vi "color_pattern_recog_server.vi"() -> ()   [LabVIEW 2014]
uses:
  <vilib>/vision/Image Controls.llb/IMAQ Image.ctl
  <vilib>/vision/NI_Vision_Development_Module.lvlib
  <vilib>/vision/driver/NI_Vision_Acquisition_Software.lvlib
panel:
  out "Number of Matches":i32
  in  "Tab Control":enum32{"Page 1", "Page 2"}(tab)
  out "bytes written":i32
  out "remote address":string
  in  "Port":u16=81 min=1025 step=1
  out "remote port":u16
  in  "Stop":bool
  out "Template":T1(plugin-control)
  in  "Image source":bool
  in  "Controls":enum32{"Page 1", "Page 2"}(tab)
  in  "Template wait":u32=1000
  in  "match wait":u32=10
  in  "Nb of Matches":i32=4
  in  "Match Mode 2":u32(ring) items=["Shift Invariant", "Rotation Invariant"]
  in  "Match Feature Mode":u32(ring) items=["Color and Shape", "Color", "Shape"]
  in  "Color Score Weight":sgl=500.0 min=0 max=1000 format="%.2f"
  in  "Minimum Contrast 2":i32=10
  in  "Color Sensitivity":u32(ring)=2 items=["Low Sensitivity", "Medium Sensitivity", "High Sensitivity"]
  in  "Search Strategy":u32(ring) items=["Conservative", "Balance", "Aggressive", "Very Aggressive"]
  in  "Minimum Score 2":sgl=700.0
  in  "Subpixel Accuracy 2":bool
  in  "File Path":path=path "C:/Users/TMRS/Desktop/image procsseing labview/Pattern matching/FuseBox/fuse01-01.jpg"
  in  "Mode select (template/match)":bool=TRUE
  in  "Template path":path=path "C:/Users/TMRS/Desktop/image procsseing labview/Pattern matching/FuseBox/fuse01-00.jpg"
  out "error":errorcluster
  out "image":T1(plugin-control)
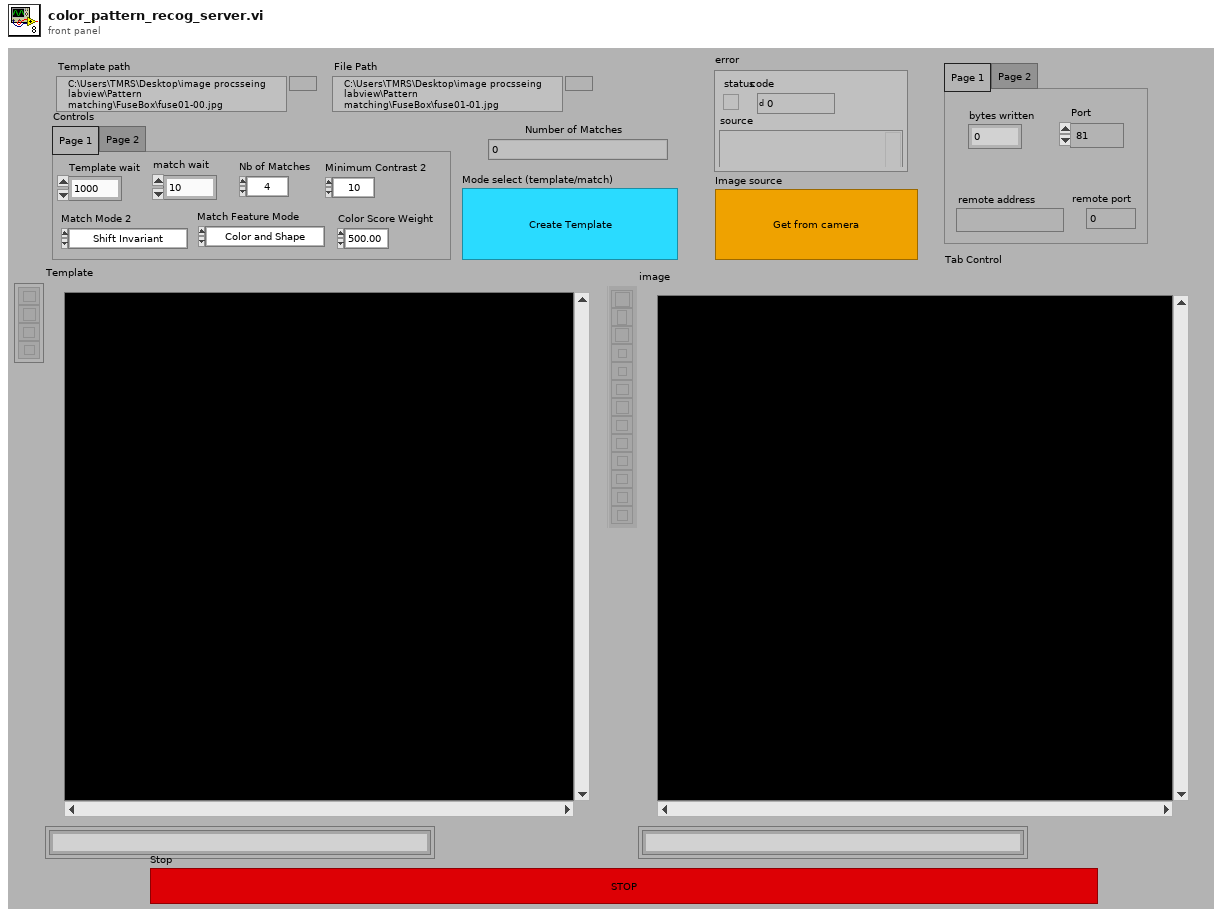
[diagram p1: front panel]
types:
  T1 = typedef "IMAQ Image.ctl" = refnum<image>
  T2 = cluster{"Position":cluster{"x":sgl, "y":sgl}, "Angle":sgl, "Scale":sgl, "Score":sgl, "Bounding Box":cluster{"x":sgl, "y":sgl}[]}[]
  T3 = cluster{"Global Rectangle":i32[], "Contours":cluster{"Contour Type":u32, "ROI Type":u32, "Points":i32[]}[]}
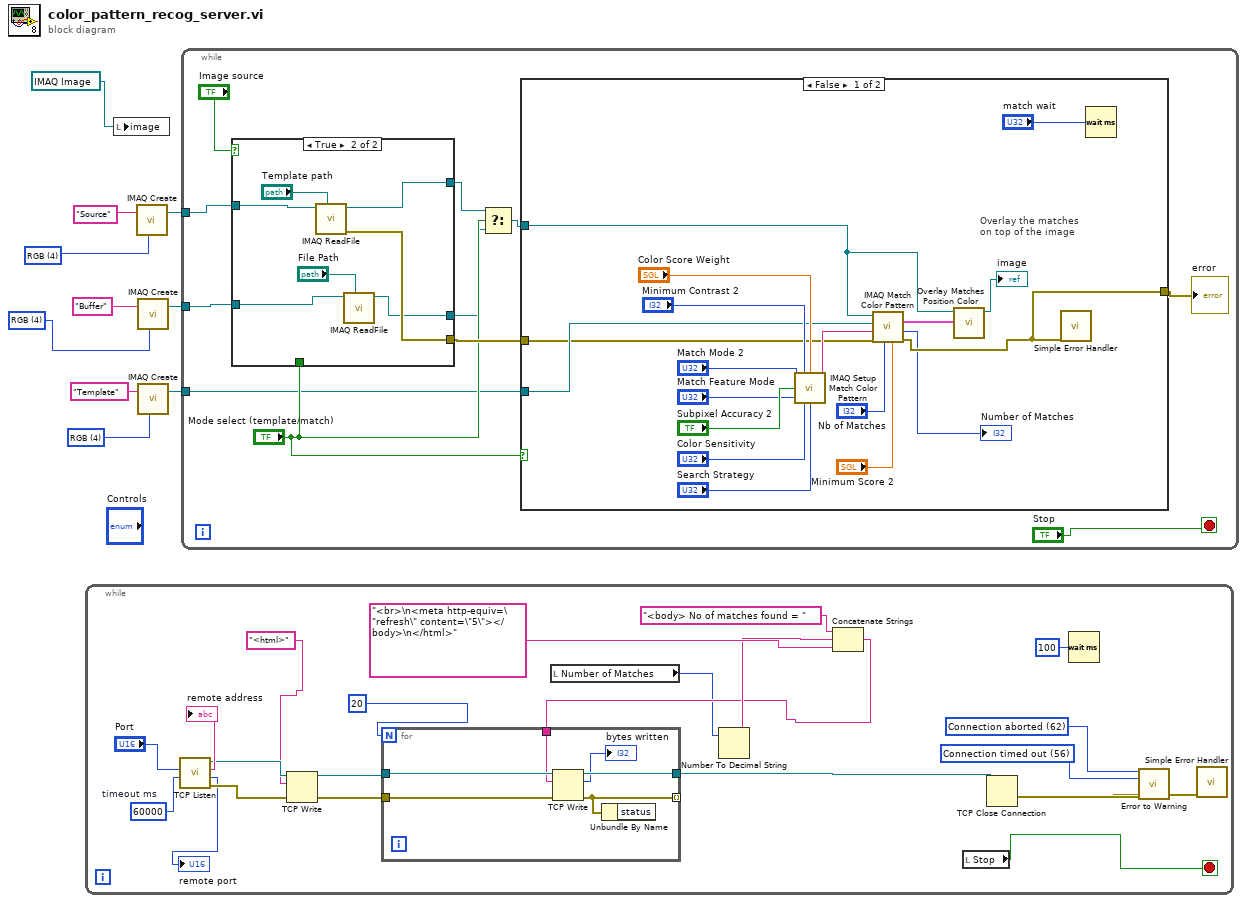
[diagram p0: block diagram]
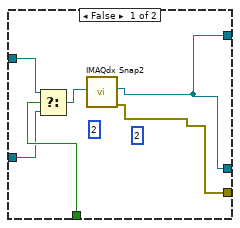
[diagram p2: hidden frame]
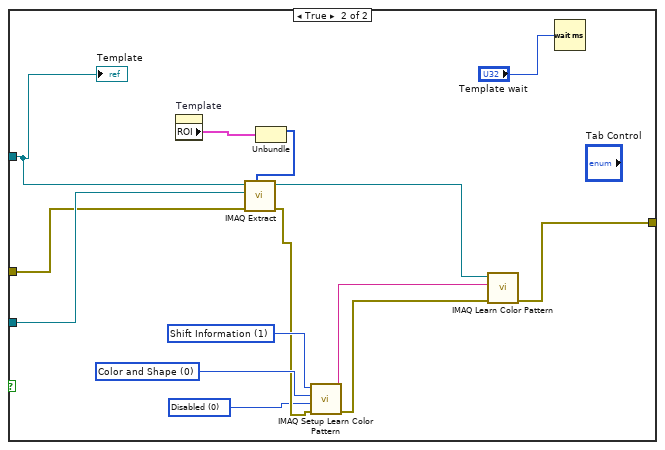
[diagram p3: hidden frame]
diagram:
  w1 = u32 4 items=["8 bits", "16 bits", "Float", "Complex", "RGB", "HSL"] ("Image Type")
  w2 = u32 4 items=["8 bits", "16 bits", "Float", "Complex", "RGB", "HSL"] ("Image Type")
  w3 = u32 4 items=["8 bits", "16 bits", "Float", "Complex", "RGB", "HSL"] ("Image Type")
  n1 = while {
    stop <- w11 stop-if-true
    w26 = 60000  # timeout ms
    w27 = 56 items=["No Error", "Argument Error", "Memory Full", "Out of Zone", "End of File", "File Already Open", "Generic File IO Error", "File Not Found", "File Permission Error", "Disk Full", "Duplicate Path", "Too Many Files Open", "Not Enabled", "Resource File Not Found", "Cannot Add Resource", "Resource Not Found", "Image Not Found", "Image Memory Error", "Pen Does Not Exist", "Config Bad Type", "Config Token Not Found", "Config Parse Error", "Config Memory Error", "Bad External Code Format", "Bad External Code Offset", "External Code Not Present", "Null Window", "Destroy Window Mixup", "Null Menu", "Print Aborted", "Bad Print Record", "Print Driver Error", "Windows Error During Print", "Memory Error During Print", "Print Dialog Error", "Generic Print Error", "Invalid Device Refnum", "Device Not Found", "Device Parameter Error", "Device Unit Error", "Can't Open Device", "Device Call Aborted", "Generic Error", "Cancelled By User", "Object ID Too Low", "Object ID Too High", "Object Not In Heap", "Unknown Heap", "Bad DefProc ID", "DefProc Not In Table", "Message Out Of Range", "Null Method", "Unknown Message", "Manager Call Not Supported", "Bad address", "Connection In progress", "Connection timed out", "Connection is already in progress", "Network attribute not supported", "Network error", "Address in use", "System out of memory", "Connection aborted", "Connection refused", "Connection is not connected", "Connection is already connected", "Connection closed", "Initialize error (interapplication manager)", "Bad occurrence", "Wait on unbound occurrence handler", "Occurrence queue overflow", "Bad path", "Semaphore not signaled", "Unrecognized type (interapplication manager)"] ("2nd Error to Convert")
    w28 = 62 items=["No Error", "Argument Error", "Memory Full", "Out of Zone", "End of File", "File Already Open", "Generic File IO Error", "File Not Found", "File Permission Error", "Disk Full", "Duplicate Path", "Too Many Files Open", "Not Enabled", "Resource File Not Found", "Cannot Add Resource", "Resource Not Found", "Image Not Found", "Image Memory Error", "Pen Does Not Exist", "Config Bad Type", "Config Token Not Found", "Config Parse Error", "Config Memory Error", "Bad External Code Format", "Bad External Code Offset", "External Code Not Present", "Null Window", "Destroy Window Mixup", "Null Menu", "Print Aborted", "Bad Print Record", "Print Driver Error", "Windows Error During Print", "Memory Error During Print", "Print Dialog Error", "Generic Print Error", "Invalid Device Refnum", "Device Not Found", "Device Parameter Error", "Device Unit Error", "Can't Open Device", "Device Call Aborted", "Generic Error", "Cancelled By User", "Object ID Too Low", "Object ID Too High", "Object Not In Heap", "Unknown Heap", "Bad DefProc ID", "DefProc Not In Table", "Message Out Of Range", "Null Method", "Unknown Message", "Manager Call Not Supported", "Bad address", "Connection In progress", "Connection timed out", "Connection is already in progress", "Network attribute not supported", "Network error", "Address in use", "System out of memory", "Connection aborted", "Connection refused", "Connection is not connected", "Connection is already connected", "Connection closed", "Initialize error (interapplication manager)", "Bad occurrence", "Wait on unbound occurrence handler", "Occurrence queue overflow", "Bad path", "Semaphore not signaled", "Unrecognized type (interapplication manager)"] ("1st Error to Convert")
    n2 = call <vilib>:"TCP Listen.vi"("timeout ms (wait forever: -1)"=w26, "port"="Port") -> ("error out"=w25:errorcluster, "remote port"=→"remote port":u16, "remote address"=→"remote address":string, "connection ID"=w20:refnum<k5>)  [unwired: 2 in, 4 out]
    n3 = TCP Write(connection ID=w20, data in="<html>") -> (connection ID out=w21:refnum<k5>)  [unwired: 1 in, 3 out]
    n4 = local read "Number of Matches"() -> (w12:i32)
    n5 = Number To Decimal String(number=w12) -> (decimal integer string=w16:string)  [unwired: 1 out]
    n6 = Concatenate Strings("<body> No of matches found = " ("data in"), w16, "<br>\n<meta http-equiv=\"refresh\" content=\"5\"></body>\n</html>" ("data in")) -> (w15:string)
    n7 = for {
      N: 20 -> [_]
      tunnel: [w37] -> _ mode=indexing
      tunnel: w21 -> [w36]
      tunnel: w25 -> [w35]
      tunnel: [w34] -> w13
      tunnel: w15 -> [w32]
      n8 = TCP Write(connection ID=w36, data in=w32, error in (no error)=w35) -> (connection ID out=w34:refnum<k5>, bytes written=→"bytes written":i32, error out=w37:errorcluster)  [unwired: 1 out]
      n9 = Unbundle By Name(w37) -> ()  [unwired: 1 out]
    }
    n10 = local read "Stop"() -> (w11:bool)
    n11 = TCP Close Connection(connection ID=w13) -> (error out=w30:errorcluster)  [unwired: 1 in, 2 out]
    n12 = Wait (ms)(milliseconds to wait=u32 100) -> ()  [unwired: 1 out]
    n13 = call <vilib>:"Error to Warning.vi"("1st Error to Convert"=w28, "2nd Error to Convert"=w27, "error in"=w30) -> ("warning out"=w29:errorcluster)  [unwired: 3 in, 9 out]
    n14 = call <vilib>:"Simple Error Handler.vi"("error in (no error)"=w29) -> ()  [unwired: 1 in, 8 out]
  }
  n15 = local write "image"(T1 refnum ("Image")) -> ()
  n16 = call "IMAQ Create"("Image Name"="Source", "Image Type"=w2) -> ("New Image"=w8:T1)  [unwired: 2 in, 2 out]
  n17 = call "IMAQ Create"("Image Name"="Buffer" ("Image 3"), "Image Type"=w1) -> ("New Image"=w7:T1)  [unwired: 2 in, 2 out]
  n18 = call "IMAQ Create"("Image Name"="Template", "Image Type"=w3) -> ("New Image"=w9:T1)  [unwired: 2 in, 2 out]
  n19 = while {
    tunnel: w9 -> [w41]
    tunnel: w8 -> [w47]
    tunnel: w7 -> [w45]
    stop <- "Stop" stop-if-true
    n20 = case shown="True" "Image source" {
      tunnel: w47 -> [w52 w61]
      tunnel: [w49 w60] -> w39
      tunnel: [w50 w59] -> w46
      tunnel: w45 -> [w53 w56]
      tunnel: [w49 w55] -> w40
      tunnel: "Mode select (template/match)" -> [w54 _]
      frame False {
        (unwired) 2 ("Step x")
        (unwired) 2 ("Step y")
        n21 = Select(t=w52, s=w54, f=w53) -> (s? t:f=w51:T1)
        n22 = call <vilib>:"IMAQdx Snap2.vi"("Image In"=w51) -> ("error out"=w50:errorcluster, "Image Out"=w49:T1)  [unwired: 8 in, 1 out]
      }
      frame True {
        n23 = call "IMAQ ReadFile"("File Path"="Template path", "Image"=w61) -> ("error out"=w59:errorcluster, "Image Out"=w60:T1)  [unwired: 3 in, 5 out]
        n24 = call "IMAQ ReadFile"("File Path"="File Path", "Image"=w56) -> ("Image Out"=w55:T1)  [unwired: 3 in, 6 out]
      }
    }
    n25 = Select(t=w39, s="Mode select (template/match)", f=w40) -> (s? t:f=w42:T1)
    n26 = case shown="False" "Mode select (template/match)" {
      tunnel: w41 -> [w67 w93]
      tunnel: w46 -> [w62 w91]
      tunnel: [w64 w84] -> w48
      tunnel: w42 -> [w66 w80]
      frame False {
        # "Overlay the matches on top of the image"
        n27 = call "IMAQ Setup Match Color Pattern"("Match Mode"="Match Mode 2", "Minimum Contrast"="Minimum Contrast 2", "Color Score Weight"="Color Score Weight", "Match Feature Mode"="Match Feature Mode", "Subpixel Accuracy"="Subpixel Accuracy 2", "Color Sensitivity"="Color Sensitivity", "Search Strategy"="Search Strategy") -> ("Match Color Pattern Setup Data"=w78:string)  [unwired: 2 in, 6 out]
        n28 = call "IMAQ Match Color Pattern"("Minimum Match Score"="Minimum Score 2", "Number of Matches Requested"="Nb of Matches", "error in (no error)"=w62, "Match Color Pattern Setup Data"=w78, "Template Image"=w67, "Image"=w66) -> ("error out"=w64:errorcluster, "Number of Matches"=→"Number of Matches":i32, "Matches"=w68:T2)  [unwired: 1 in, 2 out]
        n29 = call "Overlay Matches Position Color.vi"("Matches"=w68, "Image"=w66) -> ("Image Out"=→"image":T1)  [unwired: 9 out]
        n30 = call <vilib>:"Simple Error Handler.vi"("error in (no error)"=w64) -> ()  [unwired: 1 in, 8 out]
        n31 = Wait (ms)(milliseconds to wait="match wait") -> ()  [unwired: 1 out]
      }
      frame True {
        w82 = u32 0 items=["Disabled", "Ignore Black", "Ignore White", "Ignore Black and White"] ("Ignore Black and White")
        w85 = u32 0 items=["Color and Shape", "Color", "Shape "] ("Feature Mode")
        w87 = u32 1 items=["All", "Shift Information", "Rotation Information"] ("Learn Mode")
        n32 = property on="Template" class="ImageControl"() -> ("ROI"=w81:T3)  [unwired: 2 in, 2 out]
        n33 = Unbundle(w81) -> ("Global Rectangle"=w90:i32[])  [unwired: 1 out]
        n34 = call "IMAQ Extract"("Optional Rectangle"=w90, "error in (no error)"=w91, "Image Dst"=w93, "Image Src"=w80) -> ("error out"=w83:errorcluster, "Image Dst Out"=w86:T1)  [unwired: 2 in, 4 out]
        n35 = call "IMAQ Setup Learn Color Pattern"("error in (no error)"=w83, "Ignore Black and White"=w82, "Feature Mode"=w85, "Learn Mode"=w87) -> ("error out"=w88:errorcluster, "Learn Color Pattern Setup Data"=w89:string)  [unwired: 2 in, 4 out]
        n36 = call "IMAQ Learn Color Pattern"("error in (no error)"=w88, "Learn Color Pattern Setup Data"=w89, "Image"=w86) -> ("error out"=w84:errorcluster)  [unwired: 8 out]
        n37 = Wait (ms)(milliseconds to wait="Template wait") -> ()  [unwired: 1 out]
        "Template" <- w80
      }
    }
    "error" <- w48
  }
